vi "main.vi"(4 "force_read?":bool, 6 "custom_path":path, 7 "command":T1=enum."read_config", 8 "error in (no error)":errorcluster, 10 "index":string, 11 "config in":T2) -> (0 "error out":errorcluster, 3 "config out":T2)   [LabVIEW 2015, in "lv-config-json-indexable.lvlib"]
doc: "This VI is able to read/write configuration from all the associated modules defined in the master data cluster. It also acts as a functional global/data store in the event that no data has changed since the last write. It will self-initialize and well set an internal flag in the event an error is encountered when reading. If no command is provided, it will default to the read command."
uses:
  lv-config-json-indexable.lvlib
  public/_controls/configuration.ctl
  public/_controls/command.ctl
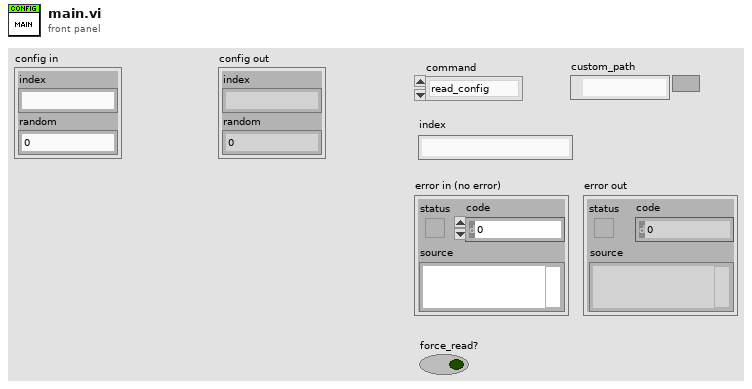
[diagram p1: front panel]
types:
  T1 = typedef "lv-config-json-indexable.lvlib/command.ctl" = enum16{"<commands>", "read_config", "write_config"}
  T2 = typedef "lv-config-json-indexable.lvlib/configuration.ctl" = cluster{"index":string, "random":dbl}
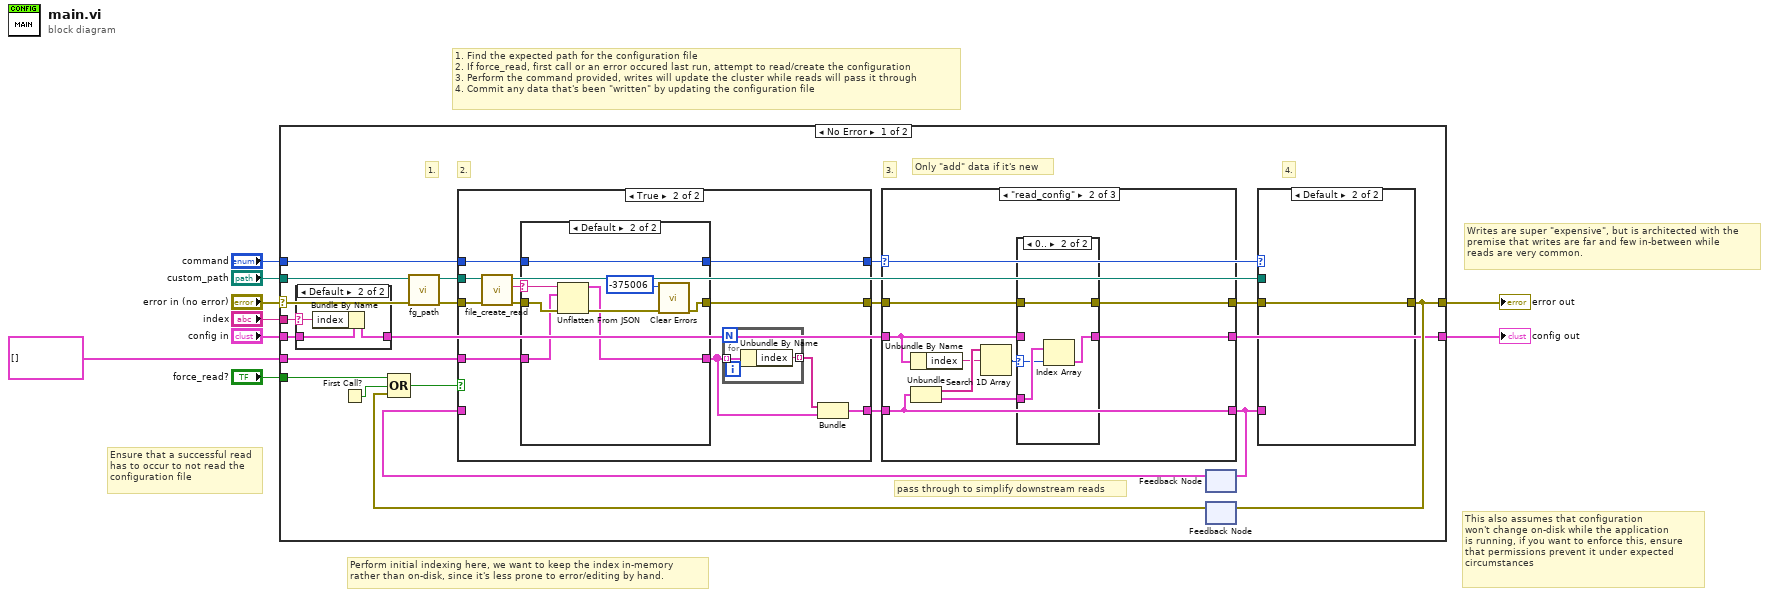
[diagram p0: block diagram]
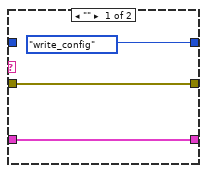
[diagram p4: hidden frame]
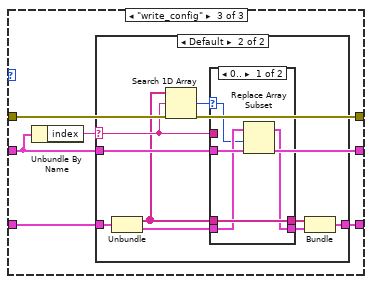
[diagram p7: hidden frame]
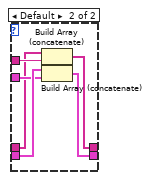
[diagram p9: hidden frame]
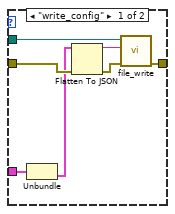
[diagram p10: hidden frame]
diagram:
  # "Perform initial indexing here, we want to keep the index in-memory\nrather than on-disk, since it's less prone to error/editing by hand."
  # "This also assumes that configuration\nwon't change on-disk while the application\nis running, if you want to enforce this, ensure\nthat permissions prevent it under expected\ncircumstances"
  # "1. Find the expected path for the configuration file\n2. If force_read, first call or an error occured last run, attempt to read/create the configuration\n3. Perform the command provided, writes will update the cluster while reads will pass it through\n4. Commit any data that's been \"written\" by updating the configuration file"
  # "Writes are super \"expensive\", but is architected with the\npremise that writes are far and few in-between while\nreads are very common."
  # "Ensure that a successful read\nhas to occur to not read the\nconfiguration file"
  n1 = case shown="No Error" "error in (no error)" {
    selector: "error in (no error)" -> [w28 w114]
    tunnel: "command" -> [w19 _]
    tunnel: [w30 w114] -> w5
    tunnel: "config in" -> [w12 _]
    tunnel: "custom_path" -> [w27 _]
    tunnel: "force_read?" -> [w25 _]
    tunnel: T2[] [] -> [w21 _]
    tunnel: [w15 _] -> w2
    tunnel: "index" -> [w11 _]
    frame No Error {
      # "pass through to simplify downstream reads"
      # "Only \"add\" data if it's new"
      # "4."
      # "3."
      # "2."
      # "1."
      n2 = case shown="Default" w11 {
        selector: w11 -> [_ w33]
        tunnel: w12 -> [w31 w34]
        tunnel: [w31 w32] -> w10
        frame "" {
        }
        frame Default {
          n3 = Bundle By Name(cluster=w34, "index"=w33) -> (w32:T2)
        }
      }
      n4 = First Call?() -> (First Call?: T/F=w26:bool)
      n5 = call "fg_path.vi"("error in (no error)"=w28, "custom_path"=w27) -> ("error out"=w22:errorcluster, "config_working"=w20:path)  [unwired: 8 in]
      n6 = feedback #1() -> (w23:cluster{string[], T2[]})  [unwired: 1 in]
      n7 = feedback #2() -> (w29:errorcluster)  [unwired: 1 in]
      n8 = Compound Arithmetic op=OR(w25, w26, w29) -> (w24:bool)
      n9 = case shown="True" w24 {
        tunnel: w23 -> [w35 _]
        tunnel: w22 -> [w37 w46]
        tunnel: w20 -> [_ w47]
        tunnel: [w37 w44] -> w14
        tunnel: w21 -> [_ w48]
        tunnel: w19 -> [w36 w43]
        tunnel: [w36 w42] -> w18
        tunnel: [w35 w38] -> w17
        frame False {
        }
        frame True {
          n10 = call "file_create_read.vi"("error in (no error)"=w46, "config_path"=w47) -> ("error out"=w45:errorcluster, "string"=w41:string)  [unwired: 8 in]
          n11 = case shown="Default" w41 {
            selector: w41 -> [_ w57]
            tunnel: w48 -> [w49 w58]
            tunnel: w45 -> [w51 w59]
            tunnel: [w51 w53] -> w44
            tunnel: w43 -> [_ w55]
            tunnel: [command."write_config" ("command") w55] -> w42
            tunnel: [w49 w54] -> w39
            frame "" {
            }
            frame Default {
              n12 = Unflatten From JSON(JSON string=w57, type and defaults=w58, error in (no error)=w59) -> (value=w54:T2[], error out=w56:errorcluster)  [unwired: 4 in]
              n13 = call <vilib>:"Clear Errors.vi"("error in (no error)"=w56, "specific error code to clear (0: all)"=-375006) -> ("error out"=w53:errorcluster)  [unwired: 4 in, 1 out]
            }
          }
          n14 = for {
            tunnel: w39 -> [w61] mode=indexing
            tunnel: [w60] -> w40 mode=indexing
            n15 = Unbundle By Name(w61) -> ("index"=w60:string)
          }
          n16 = Bundle(w40, w39) -> (w38:cluster{string[], T2[]})  [unwired: 1 in]
        }
      }
      n17 = case shown="\"read_config\"" w18 {
        tunnel: w10 -> [w63 w65 w81]
        tunnel: [w64 w73 w84] -> w16
        tunnel: w17 -> [w64 w73 w82]
        tunnel: [w63 w68 w81] -> w15
        tunnel: w14 -> [w62 w67 w80]
        tunnel: [w62 w66 w80] -> w13
        frame Default {
        }
        frame "read_config" {
          n18 = Unbundle By Name(w65) -> ("index"=w71:string)
          n19 = Unbundle(w73) -> (w72:string[], w70:T2[])
          n20 = Search 1D Array(1D array=w72, element=w71) -> (index of element=w69:i32)  [unwired: 1 in]
          n21 = case shown="0.." w69 {
            selector: w69 -> [_ w78]
            tunnel: w70 -> [_ w79]
            tunnel: [w74 w77] -> w68
            tunnel: w67 -> [w75 w76]
            tunnel: [w75 w76] -> w66
            tunnel: w65 -> [w74 _]
            frame Default {
            }
            frame 0.. {
              n22 = Index Array(array=w79, index=w78) -> (element=w77:T2)
            }
          }
        }
        frame "write_config" {
          n23 = Unbundle By Name(w81) -> ("index"=w83:string)
          n24 = case shown="Default" w83 {
            selector: w83 -> [_ w89]
            tunnel: [w85 w92] -> w84
            tunnel: w81 -> [_ w90]
            tunnel: w82 -> [w85 w87]
            frame "" {
            }
            frame Default {
              n25 = Unbundle(w87) -> (w86:string[], w88:T2[])
              n26 = Search 1D Array(1D array=w86, element=w89) -> (index of element=w94:i32)  [unwired: 1 in]
              n27 = case shown="0.." w94 {
                selector: w94 -> [w95 _]
                tunnel: w88 -> [w98 w104]
                tunnel: [w97 w102] -> w93
                tunnel: w86 -> [w99 w100]
                tunnel: [w99 w101] -> w91
                tunnel: w90 -> [w96 w103]
                tunnel: w89 -> [_ w105]
                frame 0.. {
                  n28 = Replace Array Subset(array=w98, new element=w96, index=w95) -> (w97:T2[])
                }
                frame Default {
                  n29 = Build Array (concatenate)(w100, w105) -> (w101:string[])
                  n30 = Build Array (concatenate)(w104, w103) -> (w102:T2[])
                }
              }
              n31 = Bundle(w91, w93) -> (w92:cluster{string[], T2[]})  [unwired: 1 in]
            }
          }
        }
      }
      n32 = feedback-in #1(w16) -> ()
      n33 = case shown="Default" w18 {
        tunnel: w16 -> [w109 _]
        tunnel: w13 -> [w110 w113]
        tunnel: [w107 w113] -> w30
        tunnel: w20 -> [w108 _]
        frame "write_config" {
          n34 = Unbundle(w109) -> (w106:T2[])  [unwired: 1 out]
          n35 = Flatten To JSON(anything=w106, error in (no error)=w110) -> (JSON string=w112:string, 11:w111:errorcluster)  [unwired: 1 in]
          n36 = call "file_write.vi"("error in (no error)"=w111, "string"=w112, "config_path"=w108) -> ("error out"=w107:errorcluster)  [unwired: 8 in]
        }
        frame Default {
        }
      }
      n37 = feedback-in #2(w30) -> ()
    }
    frame Error {
      # "If an error is wired in, be sure to skip over functionality to preserve the original error"
    }
  }
  "config out" <- w2
  "error out" <- w5
